vi "TWM Client Cmd Restart.vi"(7 "end of packet key":string="TWM:command:EndOfPacket", 8 "error in":errorcluster, 11 "handle":i32) -> (0 "error out":errorcluster, 3 "handle out":i32)   [LabVIEW 2020, in "TWM Client.lvlib"]
doc: "Write Reset command packet to TWM server. It will restart TWM server. This should be called just before CloseHandle of the pipe to the server."
uses:
  TWM Client.lvlib
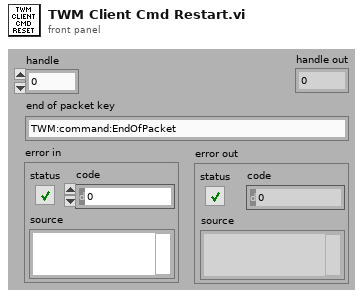
[diagram p1: front panel]
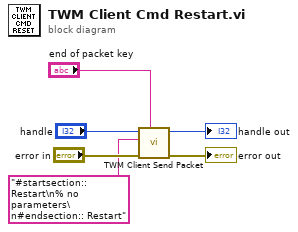
[diagram p0: block diagram]
diagram:
  n1 = call "TWM Client Send Packet.vi"("end of packet key"="end of packet key", "error in"="error in", "command string"="#startsection:: Restart\n% no parameters\n#endsection:: Restart", "handle"="handle") -> ("error out"=→"error out":errorcluster, "handle out"=→"handle out":i32)  [unwired: 6 in]
